vi "Flywheel_Linear_Velocity_To_RPM.vi"(10 "Flywheel_Radius(m)":dbl, 11 "Linear Velocity (m/s)":dbl) -> (3 "Flywheel_Velocity(RPM)":dbl)   [LabVIEW 2019]
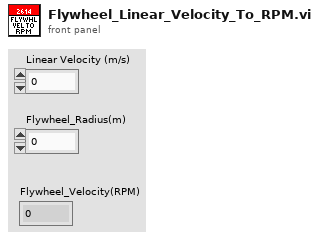
[diagram p1: front panel]
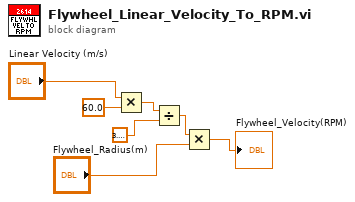
[diagram p0: block diagram]
diagram:
  n1 = Multiply(x="Linear Velocity (m/s)", y=60.0) -> (x*y=w5:dbl)
  n2 = Divide(x=w5, y=3.141592653589793) -> (x/y=w7:dbl)
  n3 = Multiply(x=w7, y="Flywheel_Radius(m)") -> (x*y=→"Flywheel_Velocity(RPM)":dbl)
